vi "yaqc_client.vi"(5 "Port":i32, 7 "host ('127.0.0.1')":string="127.0.0.1", 8 "error in (no error)":errorcluster, 10 "Python Module Path":path, 11 "Python Session In":refnum<k35>) -> (0 "error out":errorcluster, 1 "Yaqc Client":refnum<k38>, 2 "Python Module Path Out":path, 3 "Python Session Out":refnum<k35>)   [LabVIEW 2022 SP3]
doc: "Establishes a Client object associated with the daemon attached to the host and port."
uses:
  <vilib>/Utility/error.llb/Simple Error Handler.vi
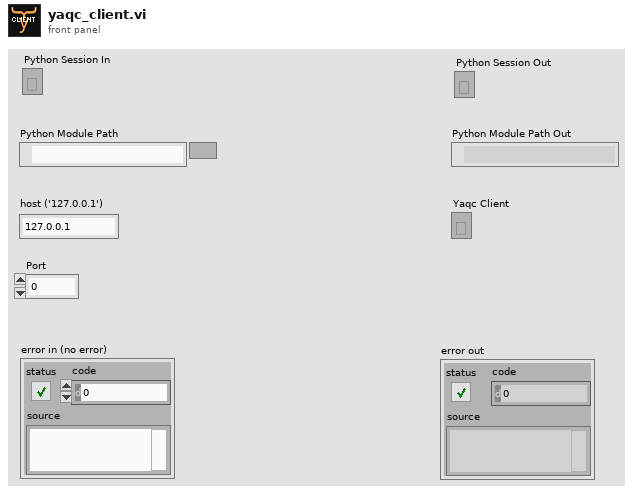
[diagram p1: front panel]
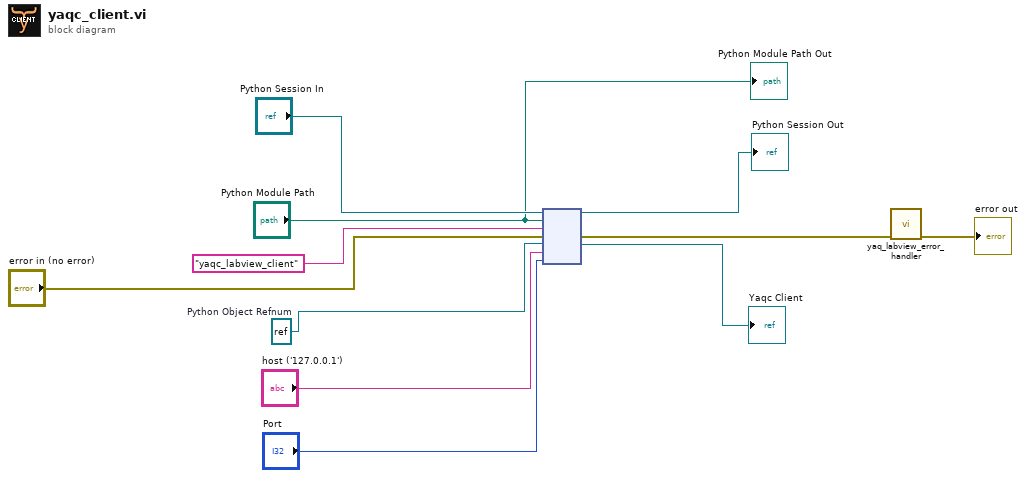
[diagram p0: block diagram]
diagram:
  w6 = refnum<k38> refnum  # Python Object Refnum
  n1 = node("Python Session In", "Python Module Path", "yaqc_labview_client" ("function name"), "error in (no error)", w6, "host ('127.0.0.1')", "Port") -> (→"Python Session Out":refnum<k35>, w1:errorcluster, →"Yaqc Client":refnum<k38>)  [unwired: 2 in, 2 out]
  n2 = call "yaq_labview_error_handler.vi"("error in (no error)"=w1) -> ("error out"=→"error out":errorcluster)  [unwired: 10 in]
  "Python Module Path Out" <- "Python Module Path"
